vi "Init Config Panel.vi"(8 "error in (no error)":errorcluster, 11 "SB App in":refnum<class "SB App.lvclass">) -> (0 "error out":errorcluster, 3 "SB App out":refnum<class "SB App.lvclass">)   [LabVIEW 2020, in "SB App.lvlib" / "SB App.lvclass"]
uses:
  SB App.lvclass
  Game Config Panel/Game Config Panel.lvclass
  C:/Program Files (x86)/National Instruments/LabVIEW 2020/vi.lib/IlluminatedG/IG OOPanel/OOPanel/Panel/Panel.lvclass
  SB App.lvclass/SB App.ctl
  <vilib>/IlluminatedG/IG OOPanel/OOPanel/Manager/Manager.lvclass
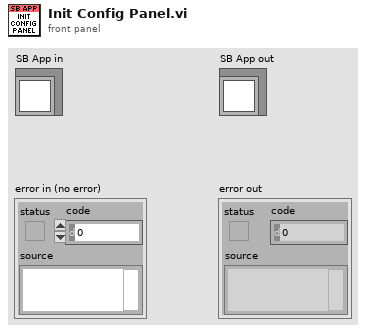
[diagram p1: front panel]
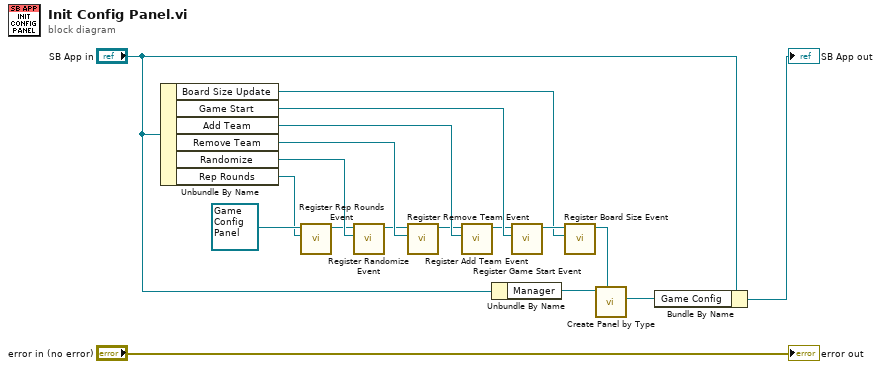
[diagram p0: block diagram]
diagram:
  n1 = Unbundle By Name("SB App in") -> ("Board Size Update"=w15:refnum<user-event>, "Game Start"=w17:refnum<user-event>, "Add Team"=w13:refnum<user-event>, "Remove Team"=w11:refnum<user-event>, "Randomize"=w9:refnum<user-event>, "Rep Rounds"=w1:refnum<user-event>)
  n2 = call "Register Rep Rounds Event.vi"("Rep Rounds"=w1, "Game Config Panel in"=refnum<class "Game Config Panel.lvclass"> refnum ("SB App.lvlib:Game Config Panel.lvclass")) -> ("Game Config Panel out"=w3:refnum<class "Game Config Panel.lvclass">)  [unwired: 8 in, 1 out]
  n3 = call "Register Randomize Event.vi"("Randomize"=w9, "Game Config Panel in"=w3) -> ("Game Config Panel out"=w10:refnum<class "Game Config Panel.lvclass">)  [unwired: 8 in, 1 out]
  n4 = call "Register Remove Team Event.vi"("Remove Team"=w11, "Game Config Panel in"=w10) -> ("Game Config Panel out"=w12:refnum<class "Game Config Panel.lvclass">)  [unwired: 8 in, 1 out]
  n5 = call "Register Add Team Event.vi"("Add Team"=w13, "Game Config Panel in"=w12) -> ("Game Config Panel out"=w14:refnum<class "Game Config Panel.lvclass">)  [unwired: 8 in, 1 out]
  n6 = Unbundle By Name("SB App in") -> ("Manager"=w7:refnum<class "Manager.lvclass">)
  n7 = call "Register Game Start Event.vi"("Game Start"=w17, "Game Config Panel in"=w14) -> ("Game Config Panel out"=w16:refnum<class "Game Config Panel.lvclass">)  [unwired: 8 in, 1 out]
  n8 = call "Register Board Size Event.vi"("Board Size Update"=w15, "Game Config Panel in"=w16) -> ("Game Config Panel out"=w5:refnum<class "Game Config Panel.lvclass">)  [unwired: 8 in, 1 out]
  n9 = call <vilib>:"Create Panel by Type.vi"("Panel Type"=w5, "Manager in"=w7) -> ("Panel"=w4:refnum<class "Game Config Panel.lvclass">)  [unwired: 7 in, 2 out]
  n10 = Bundle By Name(cluster="SB App in", "Game Config"=w4) -> (→"SB App out":refnum<class "SB App.lvclass">)
  "error out" <- "error in (no error)"
